vi "Read Boiler Constants.vi"(8 "error in":errorcluster, 11 "CFG File Refnum in":T2) -> (0 "error out":errorcluster, 2 "Boiler Configuration":T1, 3 "CFG File Refnum out":T2)   [LabVIEW 2020]
uses:
  <vilib>/Utility/config.llb/Config Data RefNum.ctl
  Boiler/Boiler Configuration.ctl
  <vilib>/Utility/config.llb/Read Key (U32).vi
  <vilib>/Utility/error.llb/Error Cluster From Error Code.vi
  <vilib>/ErrorRing/Error Ring.xnode
  <vilib>/Utility/config.llb/NI_LVConfig.lvlib
  Boiler/Boiler.lvlib
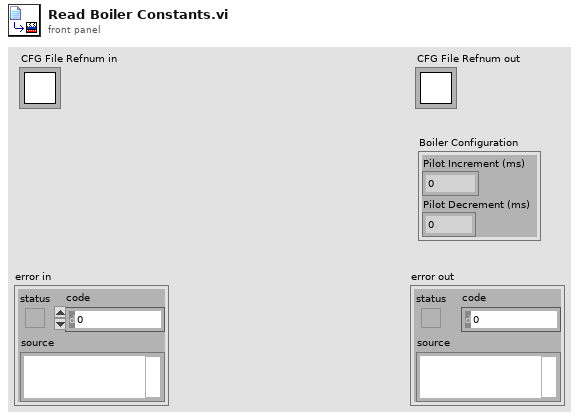
[diagram p1: front panel]
types:
  T1 = typedef "Boiler.lvlib/Boiler Configuration.ctl" = cluster{"Pilot Increment (ms)":u32, "Pilot Decrement (ms)":u32}
  T2 = typedef "NI_LVConfig.lvlib/Config Data RefNum.ctl" = refnum<k1>
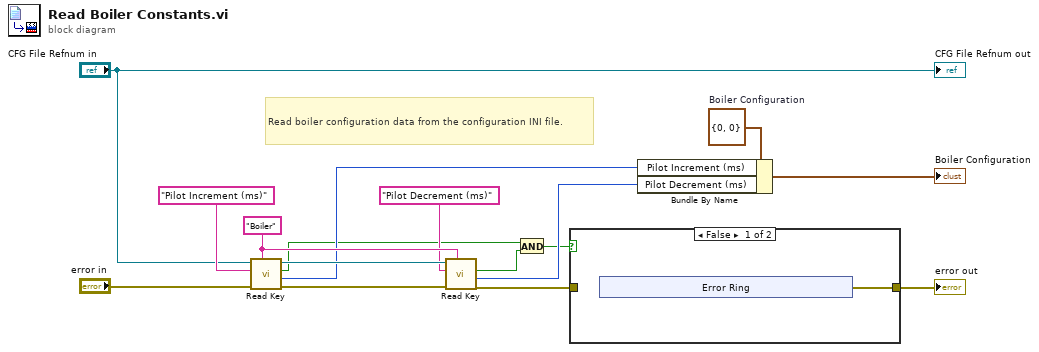
[diagram p0: block diagram]
diagram:
  w9 = T1 {"Pilot Increment (ms)"=0, "Pilot Decrement (ms)"=0}  # Boiler Configuration
  w13 = "Boiler" ("section")
  # "Read boiler configuration data from the configuration INI file."
  n1 = call-poly <vilib>:"Read Key.vi"("section"=w13, "error in (no error)"="error in", "key"="Pilot Increment (ms)", "refnum"="CFG File Refnum in") -> ("error out"=w15:errorcluster, "value"=w8:u32, "found?"=w1:bool, "refnum out"=w14:T2)  [unwired: 4 in]
  n2 = call-poly <vilib>:"Read Key.vi"("section"=w13, "error in (no error)"=w15, "key"="Pilot Decrement (ms)", "refnum"=w14) -> ("error out"=w3:errorcluster, "value"=w7:u32, "found?"=w2:bool)  [unwired: 4 in, 1 out]
  n3 = And(x=w1, y=w2) -> (x .and. y?=w5:bool)
  n4 = case shown="False" w5 {
    tunnel: [w17 w23] -> w4
    tunnel: w3 -> [_ w23]
    frame False {
      n5 = xnode "Error Ring"() -> ("error out"=w17:errorcluster)
    }
    frame True {
    }
  }
  "error out" <- w4
  n6 = Bundle By Name(cluster=w9, "Pilot Increment (ms)"=w8, "Pilot Decrement (ms)"=w7) -> (→"Boiler Configuration":T1)
  "CFG File Refnum out" <- "CFG File Refnum in"
